vi "Temperature Check.vi"(8 "error in (no error)":errorcluster, 9 "High Temp":dbl, 10 "Low Temp":dbl, 11 "Current Temperature":dbl) -> (0 "error out":errorcluster, 1 "Temperature Warning?":bool, 2 "Temperature Warning":string)   [LabVIEW 2010]
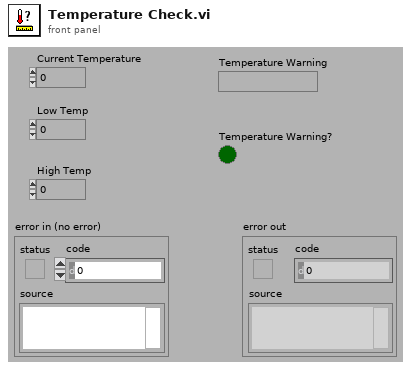
[diagram p1: front panel]
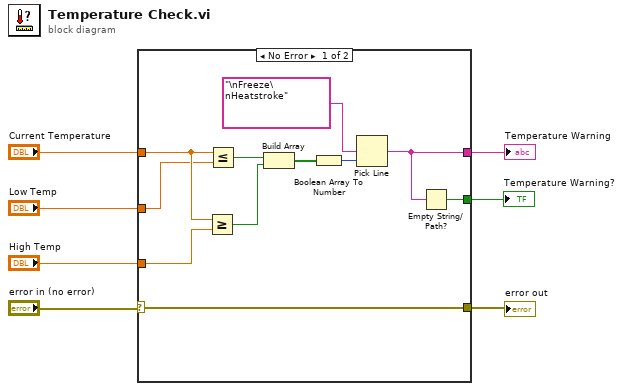
[diagram p0: block diagram]
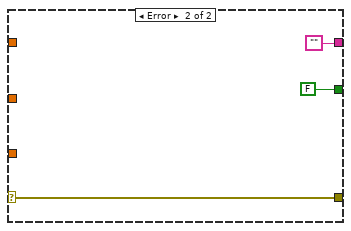
[diagram p2: hidden frame]
diagram:
  n1 = case shown="No Error" "error in (no error)" {
    selector: "error in (no error)" -> [w8 w21]
    tunnel: "Current Temperature" -> [w13 _]
    tunnel: "Low Temp" -> [w12 _]
    tunnel: "High Temp" -> [w11 _]
    tunnel: [w10 ""] -> w4
    tunnel: [w9 FALSE] -> w3
    tunnel: [w8 w21] -> w1
    frame No Error {
      n2 = Greater Or Equal?(x=w13, y=w11) -> (x >= y?=w15:bool)
      n3 = Less Or Equal?(x=w13, y=w12) -> (x <= y?=w14:bool)
      n4 = Build Array(w14, w15) -> (w16:bool[])
      n5 = Boolean Array To Number(Boolean array=w16) -> (number=w17:u32)
      n6 = Pick Line(multi-line string="\nFreeze\nHeatstroke", line index=w17) -> (output string=w10:string)  [unwired: 1 out]
      n7 = Empty String/Path?(string/path=w10) -> (empty?=w9:bool)
    }
    frame Error {
    }
  }
  "Temperature Warning" <- w4
  "Temperature Warning?" <- w3
  "error out" <- w1
